vi "GetEventHardpointMonitorInfoField.vi"(10 "Event Data":string, 11 "Cluster in":refnum<vi>) -> (3 "Array":string[](array[string]))   [LabVIEW 2016]
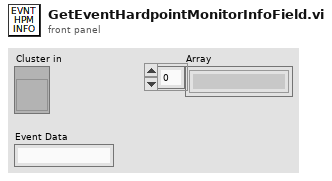
[diagram p1: front panel]
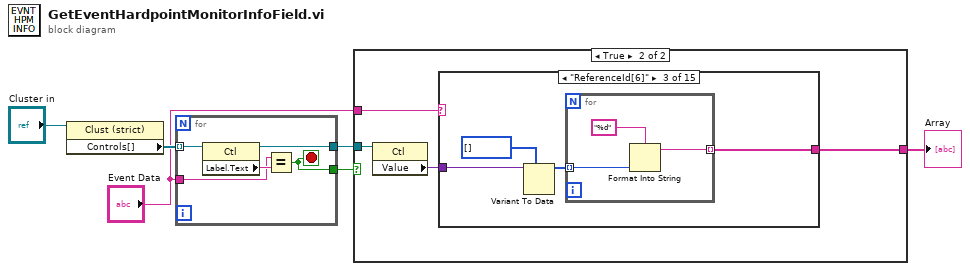
[diagram p0: block diagram]
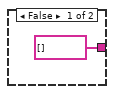
[diagram p2: hidden frame]
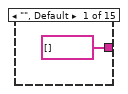
[diagram p3: hidden frame]
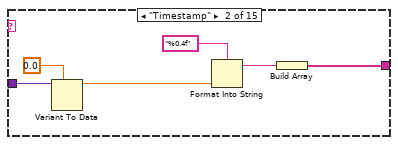
[diagram p4: hidden frame]
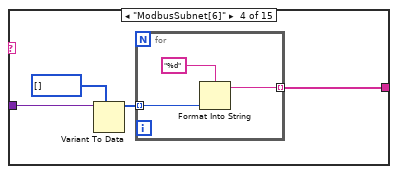
[diagram p5: hidden frame]
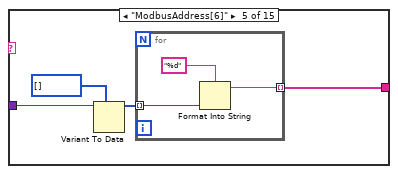
[diagram p6: hidden frame]
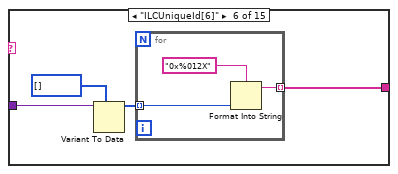
[diagram p7: hidden frame]
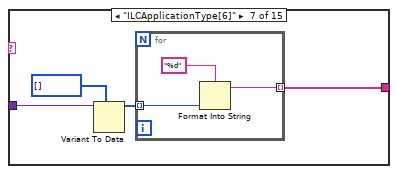
[diagram p8: hidden frame]
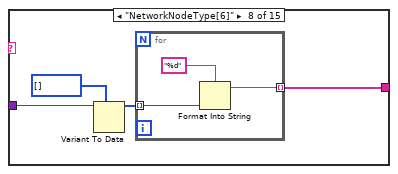
[diagram p9: hidden frame]
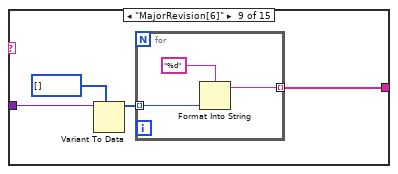
[diagram p10: hidden frame]
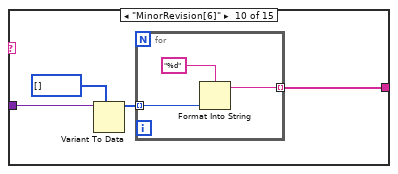
[diagram p11: hidden frame]
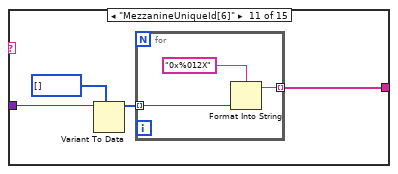
[diagram p12: hidden frame]
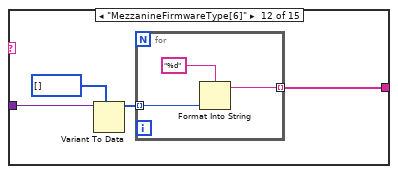
[diagram p13: hidden frame]
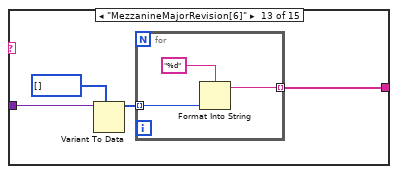
[diagram p14: hidden frame]
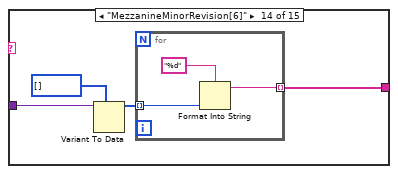
[diagram p15: hidden frame]
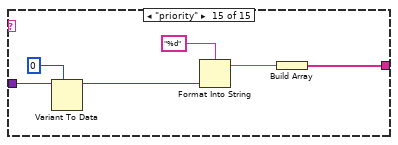
[diagram p16: hidden frame]
diagram:
  n1 = property on="Property Node" class="Clust (strict)"(reference="Cluster in") -> ("Controls[]"=w6:refnum<vi>[])  [unwired: 1 in, 2 out]
  n2 = for {
    tunnel: w6 -> [w11] mode=indexing
    tunnel: [w10] -> w3
    tunnel: "Event Data" -> [w8]
    tunnel: [w7] -> w4
    stop <- w7 stop-if-true
    n3 = property on="Property Node" class="Ctl"(reference=w11) -> (reference out=w10:refnum<vi>, "Label.Text"=w9:string)  [unwired: 1 in, 1 out]
    n4 = Equal?(x=w8, y=w9) -> (x = y?=w7:bool)
  }
  n5 = case shown="True" w4 {
    tunnel: "Event Data" -> [_ w16]
    tunnel: w3 -> [_ w15]
    tunnel: [string[] [] w13] -> w2
    frame False {
    }
    frame True {
      n6 = property on="Property Node" class="Ctl"(reference=w15) -> ("Value"=w14:variant)  [unwired: 1 in, 2 out]
      n7 = case shown="\"ReferenceId[6]\"" w16 {
        tunnel: [string[] [] w21 w24 w31 w38 w45 w52 w59 w66 w73 w80 w87 w94 w101 w111] -> w13
        tunnel: w14 -> [_ w19 w27 w34 w41 w48 w55 w62 w69 w76 w83 w90 w97 w104 w109]
        frame "", Default {
        }
        frame "Timestamp" {
          n8 = Variant To Data(type=0.0, Variant=w19) -> (data=w20:dbl)  [unwired: 1 in, 1 out]
          n9 = Format Into String(format string="%0.4f", w20) -> (resulting string=w22:string)  [unwired: 2 in, 1 out]
          n10 = Build Array(w22) -> (w21:string[])
        }
        frame "ReferenceId[6]" {
          n11 = Variant To Data(type=i16[] [], Variant=w27) -> (data=w25:i16[])  [unwired: 1 in, 1 out]
          n12 = for {
            tunnel: w25 -> [w29] mode=indexing
            tunnel: [w28] -> w24 mode=indexing
            n13 = Format Into String(format string="%d", w29) -> (resulting string=w28:string)  [unwired: 2 in, 1 out]
          }
        }
        frame "ModbusSubnet[6]" {
          n14 = Variant To Data(type=i16[] [], Variant=w34) -> (data=w32:i16[])  [unwired: 1 in, 1 out]
          n15 = for {
            tunnel: w32 -> [w36] mode=indexing
            tunnel: [w35] -> w31 mode=indexing
            n16 = Format Into String(format string="%d", w36) -> (resulting string=w35:string)  [unwired: 2 in, 1 out]
          }
        }
        frame "ModbusAddress[6]" {
          n17 = Variant To Data(type=i16[] [], Variant=w41) -> (data=w39:i16[])  [unwired: 1 in, 1 out]
          n18 = for {
            tunnel: w39 -> [w43] mode=indexing
            tunnel: [w42] -> w38 mode=indexing
            n19 = Format Into String(format string="%d", w43) -> (resulting string=w42:string)  [unwired: 2 in, 1 out]
          }
        }
        frame "ILCUniqueId[6]" {
          n20 = Variant To Data(type=i64[] [], Variant=w48) -> (data=w46:i64[])  [unwired: 1 in, 1 out]
          n21 = for {
            tunnel: w46 -> [w50] mode=indexing
            tunnel: [w49] -> w45 mode=indexing
            n22 = Format Into String(format string="0x%012X", w50) -> (resulting string=w49:string)  [unwired: 2 in, 1 out]
          }
        }
        frame "ILCApplicationType[6]" {
          n23 = Variant To Data(type=i16[] [], Variant=w55) -> (data=w53:i16[])  [unwired: 1 in, 1 out]
          n24 = for {
            tunnel: w53 -> [w57] mode=indexing
            tunnel: [w56] -> w52 mode=indexing
            n25 = Format Into String(format string="%d", w57) -> (resulting string=w56:string)  [unwired: 2 in, 1 out]
          }
        }
        frame "NetworkNodeType[6]" {
          n26 = Variant To Data(type=i16[] [], Variant=w62) -> (data=w60:i16[])  [unwired: 1 in, 1 out]
          n27 = for {
            tunnel: w60 -> [w64] mode=indexing
            tunnel: [w63] -> w59 mode=indexing
            n28 = Format Into String(format string="%d", w64) -> (resulting string=w63:string)  [unwired: 2 in, 1 out]
          }
        }
        frame "MajorRevision[6]" {
          n29 = Variant To Data(type=i16[] [], Variant=w69) -> (data=w67:i16[])  [unwired: 1 in, 1 out]
          n30 = for {
            tunnel: w67 -> [w71] mode=indexing
            tunnel: [w70] -> w66 mode=indexing
            n31 = Format Into String(format string="%d", w71) -> (resulting string=w70:string)  [unwired: 2 in, 1 out]
          }
        }
        frame "MinorRevision[6]" {
          n32 = Variant To Data(type=i16[] [], Variant=w76) -> (data=w74:i16[])  [unwired: 1 in, 1 out]
          n33 = for {
            tunnel: w74 -> [w78] mode=indexing
            tunnel: [w77] -> w73 mode=indexing
            n34 = Format Into String(format string="%d", w78) -> (resulting string=w77:string)  [unwired: 2 in, 1 out]
          }
        }
        frame "MezzanineUniqueId[6]" {
          n35 = Variant To Data(type=i64[] [], Variant=w83) -> (data=w81:i64[])  [unwired: 1 in, 1 out]
          n36 = for {
            tunnel: w81 -> [w85] mode=indexing
            tunnel: [w84] -> w80 mode=indexing
            n37 = Format Into String(format string="0x%012X", w85) -> (resulting string=w84:string)  [unwired: 2 in, 1 out]
          }
        }
        frame "MezzanineFirmwareType[6]" {
          n38 = Variant To Data(type=i16[] [], Variant=w90) -> (data=w88:i16[])  [unwired: 1 in, 1 out]
          n39 = for {
            tunnel: w88 -> [w92] mode=indexing
            tunnel: [w91] -> w87 mode=indexing
            n40 = Format Into String(format string="%d", w92) -> (resulting string=w91:string)  [unwired: 2 in, 1 out]
          }
        }
        frame "MezzanineMajorRevision[6]" {
          n41 = Variant To Data(type=i16[] [], Variant=w97) -> (data=w95:i16[])  [unwired: 1 in, 1 out]
          n42 = for {
            tunnel: w95 -> [w99] mode=indexing
            tunnel: [w98] -> w94 mode=indexing
            n43 = Format Into String(format string="%d", w99) -> (resulting string=w98:string)  [unwired: 2 in, 1 out]
          }
        }
        frame "MezzanineMinorRevision[6]" {
          n44 = Variant To Data(type=i16[] [], Variant=w104) -> (data=w102:i16[])  [unwired: 1 in, 1 out]
          n45 = for {
            tunnel: w102 -> [w106] mode=indexing
            tunnel: [w105] -> w101 mode=indexing
            n46 = Format Into String(format string="%d", w106) -> (resulting string=w105:string)  [unwired: 2 in, 1 out]
          }
        }
        frame "priority" {
          n47 = Variant To Data(type=0, Variant=w109) -> (data=w110:i32)  [unwired: 1 in, 1 out]
          n48 = Format Into String(format string="%d", w110) -> (resulting string=w112:string)  [unwired: 2 in, 1 out]
          n49 = Build Array(w112) -> (w111:string[])
        }
      }
    }
  }
  "Array" <- w2
